vi "Quey 2400 set voltage.vi"(8 "错误输入（无错误）":errorcluster, 11 "VISA资源名称":refnum<visa-resource-name>) -> (0 "错误输出":errorcluster, 2 "Set Voltage":dbl)   [LabVIEW 2019, in "User lib.lvlib"]
uses:
  User lib.lvlib
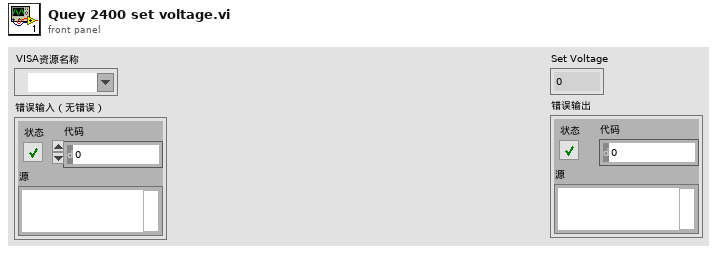
[diagram p1: front panel]
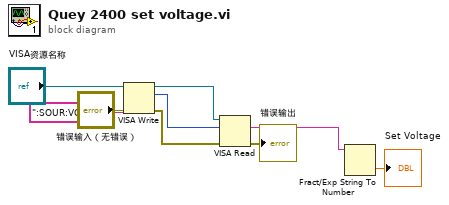
[diagram p0: block diagram]
diagram:
  n1 = VISA Write(VISA resource name="VISA资源名称", write buffer=":SOUR:VOLT?" ("写入缓冲区"), error in (no error)="错误输入（无错误）") -> (VISA resource name out=w7:refnum<visa-resource-name>, return count=w5:u32, error out=w6:errorcluster)
  n2 = VISA Read(VISA resource name=w7, byte count=w5, error in (no error)=w6) -> (read buffer=w4:string, error out=→"错误输出":errorcluster)  [unwired: 2 out]
  n3 = Fract/Exp String To Number(string=w4) -> (number=→"Set Voltage":dbl)  [unwired: 3 in, 1 out]
